vi "Close.vi"(8 "error in (no error)":errorcluster, 11 "WebSocket Client in":refnum<class "WebSocket Client.lvclass">) -> (0 "error out":errorcluster, 3 "WebSocket Client out":refnum<class "WebSocket Client.lvclass">)   [LabVIEW 2020, in "HTTP Server.lvlib" / "WebSocket Client.lvclass"]
uses:
  WebSocket Client.lvclass
  WebSocket Client.lvclass/WebSocket Client.ctl
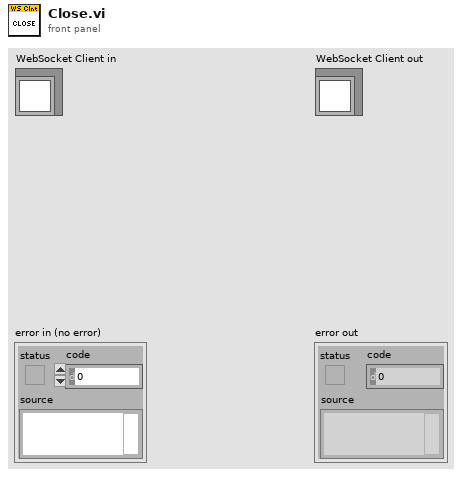
[diagram p1: front panel]
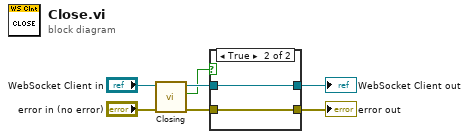
[diagram p0: block diagram]
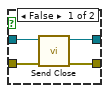
[diagram p2: hidden frame]
diagram:
  n1 = call "Closing.vi"("error in (no error)"="error in (no error)", "WebSocket Client in"="WebSocket Client in") -> ("error out"=w5:errorcluster, "Closing"=w4:bool, "WebSocket Client out"=w6:refnum<class "WebSocket Client.lvclass">)  [unwired: 7 in]
  n2 = case shown="True" w4 {
    tunnel: w6 -> [w11 w13]
    tunnel: w5 -> [w10 w12]
    tunnel: [w9 w13] -> w3
    tunnel: [w8 w12] -> w2
    frame False {
      n3 = call "Send Close.vi"("error in (no error)"=w10, "WebSocket Client in"=w11) -> ("error out"=w8:errorcluster, "WebSocket Client out"=w9:refnum<class "WebSocket Client.lvclass">)  [unwired: 8 in]
    }
    frame True {
    }
  }
  "error out" <- w2
  "WebSocket Client out" <- w3
